vi "读取产品参数信息-CCD1CCD2.vi"(8 "错误输入（无错误）":errorcluster, 11 "LoadProductName":string) -> (0 "错误输出":errorcluster)   [LabVIEW 2017]
uses:
  Global System.vi
panel:
  out "连接的字符串":string
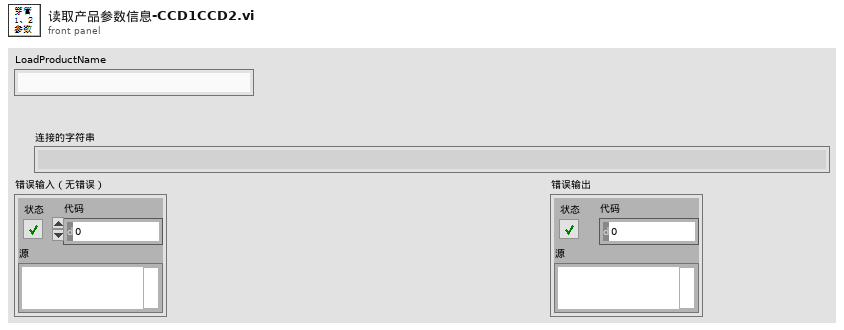
[diagram p1: front panel]
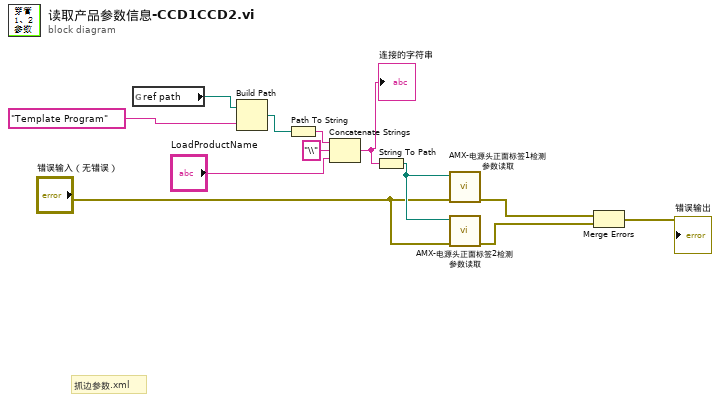
[diagram p0: block diagram]
diagram:
  # "抓边参数.xml"
  n1 = global read "Global System.vi" "ref path"() -> (w12:path)
  n2 = Build Path(base path=w12, name or relative path="Template Program" ("名称或相对路径")) -> (appended path=w10:path)
  n3 = Path To String(path=w10) -> (string=w9:string)
  n4 = Concatenate Strings(w9, "\\" ("字符串"), "LoadProductName") -> (w6:string)
  "连接的字符串" <- w6
  n5 = String To Path(string=w6) -> (path=w2:path)
  n6 = call "AMX-电源头正面标签1检测参数读取.vi"("error in (no error)"="错误输入（无错误）", "基路径"=w2) -> ("error out"=w5:errorcluster)  [unwired: 5 in, 3 out]
  n7 = call "AMX-电源头正面标签2检测参数读取.vi"("error in (no error)"="错误输入（无错误）", "基路径"=w2) -> ("error out"=w3:errorcluster)  [unwired: 5 in, 3 out]
  n8 = Merge Errors(w5, w3) -> (→"错误输出":errorcluster)
